vi "notificationhandler.vi"(0 "HGF_DSCMonitor in":refnum<class "HGF_DSCMonitor.lvclass">, 2 "notification":T1, 5 "error in (no error)":errorcluster) -> (14 "HGF_DSCMonitor out":refnum<class "HGF_DSCMonitor.lvclass">, 19 "error out":errorcluster)   [LabVIEW 2009]
uses:
  HGF_DSCMonitor.lvclass
  HGF_BaseClasses/HGF_NetworkVisitor/HGF_NetworkVisitor.lvclass
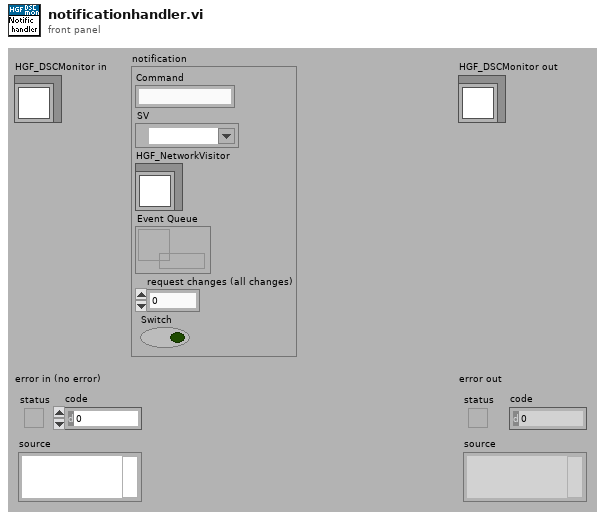
[diagram p1: front panel]
types:
  T1 = cluster{"Command":string, "SV":refnum<k21>, "HGF_NetworkVisitor":refnum<class "HGF_NetworkVisitor.lvclass">, "Event Queue":refnum<queue>, "request changes (all changes)":u16, "Switch":bool}
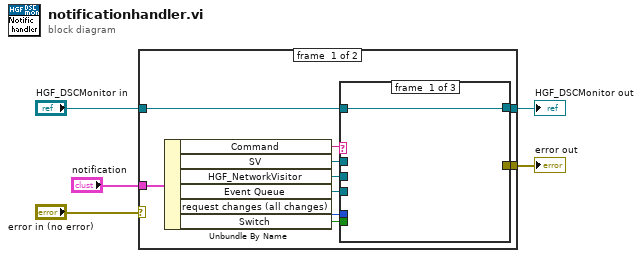
[diagram p0: block diagram]
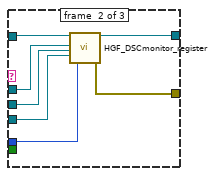
[diagram p2: hidden frame]
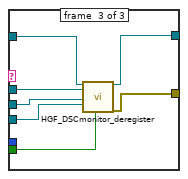
[diagram p3: hidden frame]
diagram:
  n1 = case shown="No Error" "error in (no error)" {
    selector: "error in (no error)" -> [_ w32]
    tunnel: [w8 w32] -> w4
    tunnel: [w9 w31] -> w2
    tunnel: "HGF_DSCMonitor in" -> [w13 w31]
    tunnel: "notification" -> [w15 _]
    frame #0 {
      n2 = Unbundle By Name(w15) -> ("Command"=w14:string, "SV"=w12:refnum<k21>, "HGF_NetworkVisitor"=w11:refnum<class "HGF_NetworkVisitor.lvclass">, "Event Queue"=w10:refnum<queue>, "request changes (all changes)"=w7:u16, "Switch"=w6:bool)
      n3 = case shown="\"deregister\"" w14 {
        tunnel: w13 -> [w16 w23 w30]
        tunnel: w12 -> [_ w22 w29]
        tunnel: w11 -> [_ w21 w28]
        tunnel: w10 -> [_ w20 w27]
        tunnel: [w16 w19 w24] -> w9
        tunnel: [_ w18 w25] -> w8
        tunnel: w7 -> [_ w17 _]
        tunnel: w6 -> [_ _ w26]
        frame #0 {
        }
        frame #1 {
          n4 = call "HGF_DSCmonitor_register.vi"("HGF_DSCMonitor in"=w23, "SV"=w22, "HGF_NetworkVisitor"=w21, "Event Queue"=w20, "request changes (all changes)"=w17) -> ("HGF_DSCMonitor out"=w19:refnum<class "HGF_DSCMonitor.lvclass">, "error out"=w18:errorcluster)  [unwired: 1 in, 12 out]
        }
        frame #2 {
          n5 = call "HGF_DSCmonitor_deregister.vi"("HGF_DSCMonitor in"=w30, "SV"=w29, "HGF_NetworkVisitor"=w28, "Event Queue"=w27, "Rem SV/Visitor from List"=w26) -> ("HGF_DSCMonitor out"=w24:refnum<class "HGF_DSCMonitor.lvclass">, "error out"=w25:errorcluster)  [unwired: 1 in, 12 out]
        }
      }
    }
    frame #1 {
    }
  }
  "error out" <- w4
  "HGF_DSCMonitor out" <- w2
